vi "main.vi"() -> ()   [LabVIEW 2018]
panel:
  in  "Tabbladen":enum32{"Start", "Settings", "Debug"}(tab)
  in  "MCU port":refnum<visa-resource-name>="COM10"
  in  "Odrive port":refnum<visa-resource-name>="COM9"
  in  "stop":bool
  in  "min out":dbl
  in  "max out":dbl=10.0
  in  "min in":dbl
  in  "max in":dbl=10.0 format="%#.3g"
  in  "control mode":T1(ring)
  in  "sensor select":T2(ring)=enum."slider"
  out "input":dbl
  out "output":dbl
  in  "output status":bool
  in  "slider":dbl(slide) scale=0.0..10.0
  in  "numeric":dbl
  in  "reboot ODrive":bool
  in  "MCU baud rate":u32=9600
  in  "velocity limit":dbl=10.0
  in  "max motor current":dbl=10.0
  out "MCU sluiterror":errorcluster
  out "motorsturing sluiterror":errorcluster
  out "motorsturing verzenderror":errorcluster
  out "MCU leeserror":errorcluster
  out "motorsturing connectie error":errorcluster
  out "MCU connectie error":errorcluster
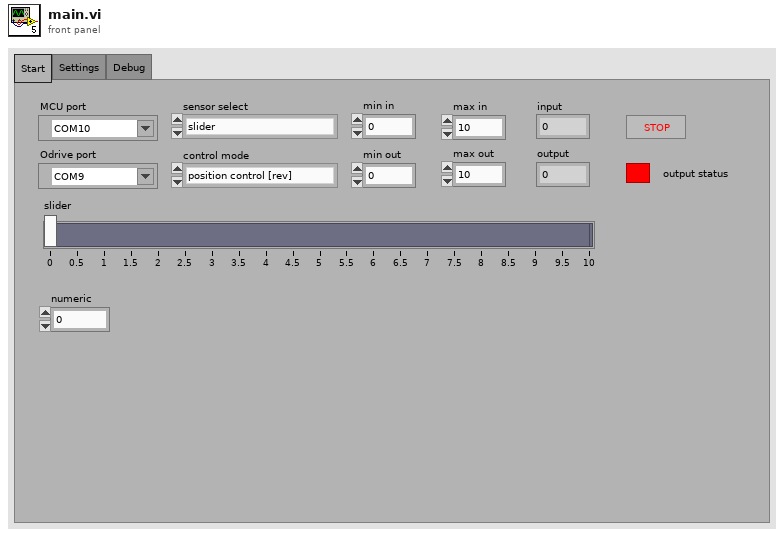
[diagram p1: front panel]
types:
  T1 = enum16{"position control [rev]", "velocity control [rev/s]", "torque control [Nm]"}
  T2 = enum16{"loadcell", "thermistor", "potentiometer", "slider", "numeric"}
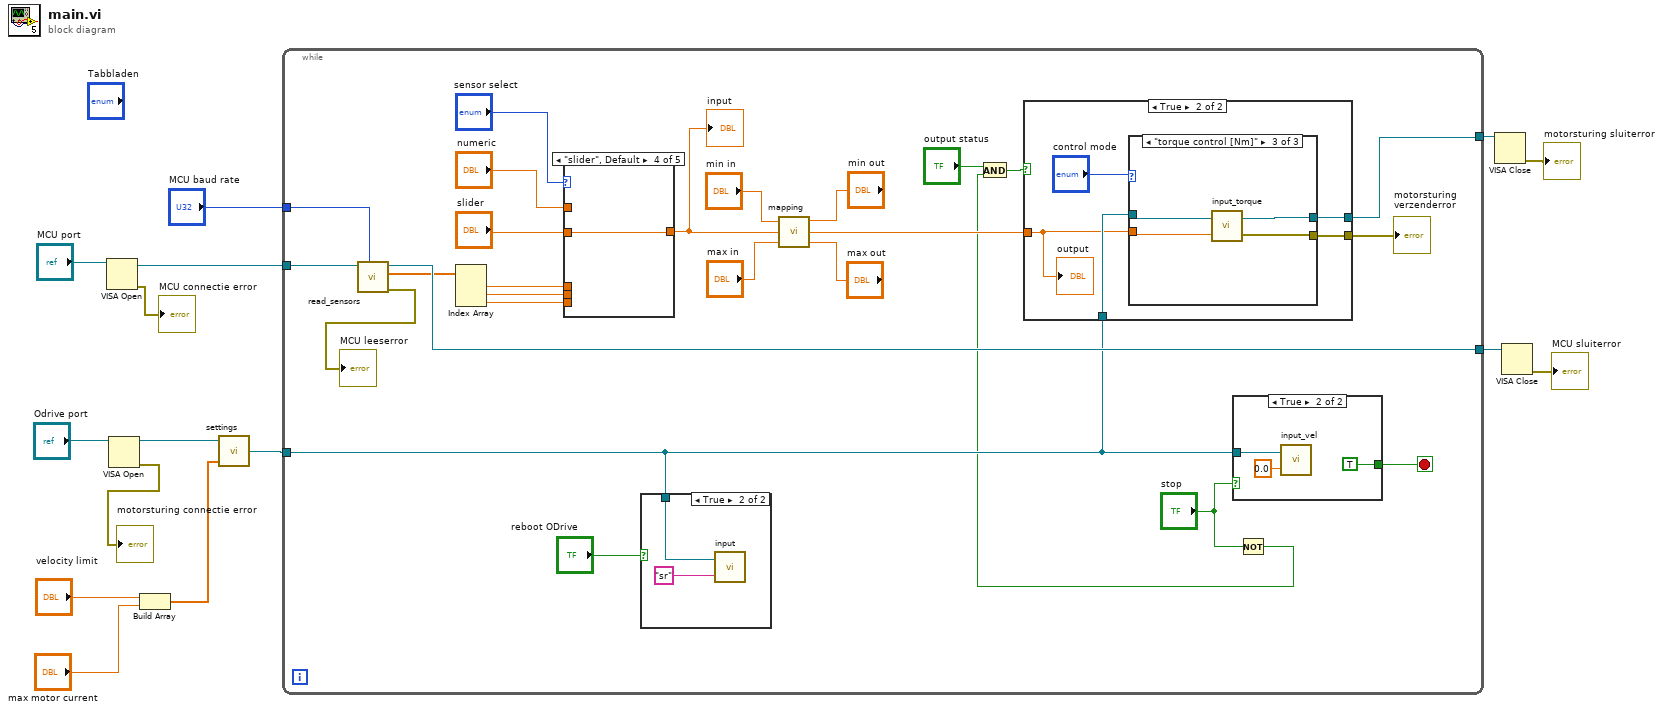
[diagram p0: block diagram]
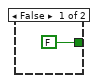
[diagram p2: hidden frame]
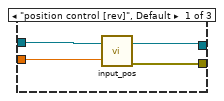
[diagram p5: hidden frame]
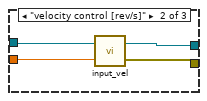
[diagram p6: hidden frame]
diagram:
  n1 = VISA Open(VISA resource name="MCU port") -> (VISA resource name=w14:refnum<visa-resource-name>, error out=→"MCU connectie error":errorcluster)  [unwired: 4 in]
  n2 = VISA Open(VISA resource name="Odrive port") -> (VISA resource name=w2:refnum<visa-resource-name>, error out=→"motorsturing connectie error":errorcluster)  [unwired: 4 in]
  n3 = Build Array("velocity limit", "max motor current") -> (w6:dbl[])
  n4 = call "settings.vi"("values"=w6, "sturing in"=w2) -> ("sturing out"=w3:refnum<visa-resource-name>)  [unwired: 3 in]
  n5 = while {
    tunnel: w3 -> [w18]
    tunnel: [w28] -> w9
    tunnel: w14 -> [w40]
    tunnel: [w41] -> w15
    tunnel: "MCU baud rate" -> [w24]
    stop <- w23 stop-if-true
    n6 = call "read_sensors.vi"("baud rate"=w24, "VISA COM"=w40) -> ("error out"=→"MCU leeserror":errorcluster, "sensor array"=w39:dbl[], "VISA COM"=w41:refnum<visa-resource-name>)  [unwired: 7 in]
    n7 = Index Array(array=w39) -> (element #1=w35:dbl, element #2=w34:dbl, element #3=w33:dbl)  [unwired: 3 in]
    n8 = case shown="\"slider\", Default" "sensor select" {
      tunnel: [w65 w66 w67 w68 w69] -> w36
      tunnel: w35 -> [w65 _ _ _ _]
      tunnel: w34 -> [_ w66 _ _ _]
      tunnel: w33 -> [_ _ w67 _ _]
      tunnel: "slider" -> [_ _ _ w68 _]
      tunnel: "numeric" -> [_ _ _ _ w69]
      frame "loadcell" {
      }
      frame "thermistor" {
      }
      frame "potentiometer" {
      }
      frame "slider", Default {
      }
      frame "numeric" {
      }
    }
    "input" <- w36
    n9 = case shown="True" "reboot ODrive" {
      tunnel: w18 -> [_ w47]
      frame False {
      }
      frame True {
        n10 = call "input.vi"("commando"="sr", "VISA in"=w47) -> ()  [unwired: 2 out]
      }
    }
    n11 = call "mapping.vi"("max out"="max out", "min out"="min out", "max in"="max in", "in"=w36, "min in"="min in") -> ("out"=w29:dbl)
    n12 = case shown="True" "stop" {
      tunnel: w18 -> [_ w45]
      tunnel: [FALSE TRUE] -> w23
      frame False {
      }
      frame True {
        n13 = call "input_vel.vi"("input"=0.0, "odrive"=w45) -> ()  [unwired: 2 out]
      }
    }
    n14 = Not(x="stop") -> (.not. x?=w16:bool)
    n15 = And(x="output status", y=w16) -> (x .and. y?=w21:bool)
    n16 = case shown="True" w21 {
      tunnel: w18 -> [_ w52]
      tunnel: w29 -> [_ w48]
      tunnel: [_ w51] -> w28
      tunnel: [_ w50] -> w22
      frame False {
      }
      frame True {
        n17 = case shown="\"torque control [Nm]\"" "control mode" {
          tunnel: w52 -> [w55 w60 w63]
          tunnel: w48 -> [w56 w59 w64]
          tunnel: [w54 w58 w62] -> w51
          tunnel: [w53 w57 w61] -> w50
          frame "position control [rev]", Default {
            n18 = call "input_pos.vi"("positie"=w56, "VISA in"=w55) -> ("error out"=w53:errorcluster, "VISA out"=w54:refnum<visa-resource-name>)
          }
          frame "velocity control [rev/s]" {
            n19 = call "input_vel.vi"("input"=w59, "odrive"=w60) -> ("error out"=w57:errorcluster, "VISA resource name out"=w58:refnum<visa-resource-name>)
          }
          frame "torque control [Nm]" {
            n20 = call "input_torque.vi"("input"=w64, "odrive"=w63) -> ("error out"=w61:errorcluster, "VISA resource name out"=w62:refnum<visa-resource-name>)
          }
        }
        "output" <- w48
      }
    }
    "motorsturing verzenderror" <- w22
  }
  n21 = VISA Close(VISA resource name=w9) -> (error out=→"motorsturing sluiterror":errorcluster)  [unwired: 1 in]
  n22 = VISA Close(VISA resource name=w15) -> (error out=→"MCU sluiterror":errorcluster)  [unwired: 1 in]
